vi "DoubleProducer_ConsumerGraphing.vi"() -> ()   [LabVIEW 2019]
panel:
  out "XY Graph":cluster{cluster{dbl, dbl}[]}[](graph)
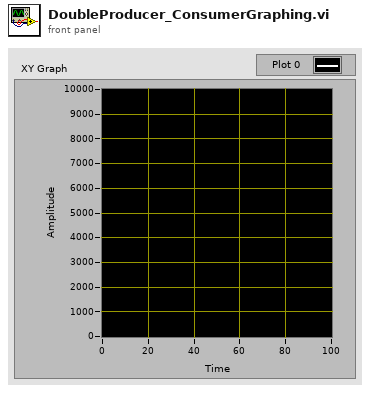
[diagram p1: front panel]
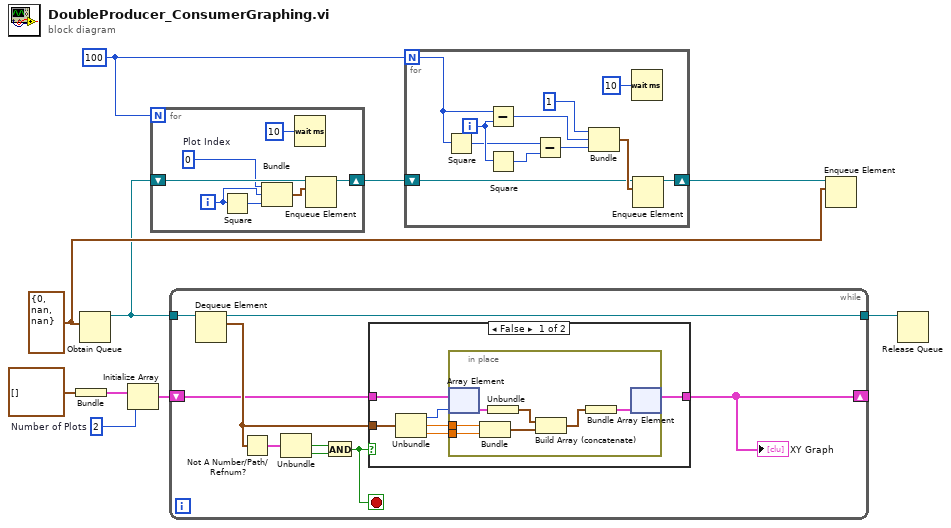
[diagram p0: block diagram]
diagram:
  w2 = 2  # Number of Plots
  w7 = cluster{i32, dbl, dbl} {0, nan, nan} ("output cluster")
  w10 = 100
  n1 = Bundle(cluster{dbl, dbl}[] []) -> (w3:cluster{cluster{dbl, dbl}[]})  [unwired: 1 in]
  n2 = Obtain Queue(element data type=w7) -> (queue out=w6:refnum<queue>)  [unwired: 4 in, 2 out]
  n3 = Initialize Array(w3, w2) -> (w1:cluster{cluster{dbl, dbl}[]}[])
  n4 = for {
    N: w10 -> [_]
    shift-right: [w12] -> w9
    shift-left: w6 -> [w13]
    i -> [w17]
    w11 = 0  # Plot Index
    n5 = Square(x=w17) -> (x^2=w16:i32)
    n6 = Bundle("Plot Index"=w11, w17, w16) -> (w15:cluster{"Plot Index":i32, i32, i32})  [unwired: 1 in]
    n7 = Wait (ms)(milliseconds to wait=u32 10) -> ()  [unwired: 1 out]
    n8 = Enqueue Element(queue=w13, element=w15) -> (queue out=w12:refnum<queue>)  [unwired: 2 in, 2 out]
  }
  n9 = while {
    tunnel: w6 -> [w26]
    shift-right: [w20] -> _
    shift-left: w1 -> [w21]
    tunnel: [w19] -> w5
    stop <- w23 stop-if-true
    n10 = Dequeue Element(queue=w26) -> (queue out=w19:refnum<queue>, element=w22:cluster{i32, dbl, dbl})  [unwired: 2 in, 2 out]
    n11 = Not A Number/Path/Refnum?(number/path/refnum=w22) -> (NaN/Path/Refnum?=w25:cluster{bool, bool, bool})
    n12 = Unbundle(w25) -> (w24:bool, w18:bool)  [unwired: 1 out]
    n13 = And(x=w24, y=w18) -> (x .and. y?=w23:bool)
    n14 = case shown="False" w23 {
      tunnel: w22 -> [w32 _]
      tunnel: [w27 w40] -> w20
      tunnel: w21 -> [w31 w40]
      frame False {
        n15 = Unbundle(w32) -> (w30:i32, w29:dbl, w28:dbl)
        n16 = in-place {
          in-place-border: w29 -> [w38]
          in-place-border: w28 -> [w37]
          n17 = in-place-array #1(w31, w30) -> (w39:cluster{cluster{dbl, dbl}[]})
          n18 = Bundle(w38, w37) -> (w35:cluster{dbl, dbl})  [unwired: 1 in]
          n19 = Unbundle(w39) -> (w36:cluster{dbl, dbl}[])
          n20 = Build Array (concatenate)(w36, w35) -> (w34:cluster{dbl, dbl}[])
          n21 = Bundle(w34) -> (w33:cluster{cluster{dbl, dbl}[]})  [unwired: 1 in]
          n22 = in-place-array #1(w33) -> (w27:cluster{cluster{dbl, dbl}[]}[])  [unwired: 1 out]
        }
      }
      frame True {
      }
    }
    "XY Graph" <- w20
  }
  n23 = for {
    N: w10 -> [w44]
    shift-right: [w48] -> w8
    shift-left: w9 -> [w49]
    i -> [w47]
    n24 = Square(x=w44) -> (x^2=w45:i32)
    n25 = Subtract(x=w44, y=w47) -> (x-y=w46:i32)
    n26 = Square(x=w47) -> (x^2=w43:i32)
    n27 = Subtract(x=w45, y=w43) -> (x-y=w42:i32)
    n28 = Bundle(1, w46, w42) -> (w51:cluster{i32, i32, i32})  [unwired: 1 in]
    n29 = Wait (ms)(milliseconds to wait=u32 10) -> ()  [unwired: 1 out]
    n30 = Enqueue Element(queue=w49, element=w51) -> (queue out=w48:refnum<queue>)  [unwired: 2 in, 2 out]
  }
  n31 = Enqueue Element(queue=w8, element=w7) -> ()  [unwired: 2 in, 3 out]
  n32 = Release Queue(queue=w5) -> ()  [unwired: 2 in, 3 out]
